vi "Wrap Phase.vi"(11 "input phase":dbl) -> (3 "wrapped phase":dbl)   [LabVIEW 2019, in "DSP.lvclass"]
uses:
  DSP.lvclass
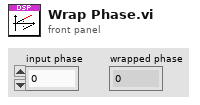
[diagram p1: front panel]
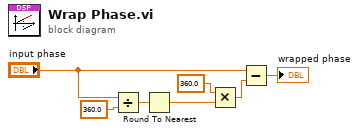
[diagram p0: block diagram]
diagram:
  n1 = Divide(x="input phase", y=360.0 ("x")) -> (x/y=w4:dbl)
  n2 = Round To Nearest(number=w4) -> (nearest integer value=w5:dbl)
  n3 = Multiply(x=360.0, y=w5) -> (x*y=w6:dbl)
  n4 = Subtract(x="input phase", y=w6) -> (x-y=→"wrapped phase":dbl)
